vi "Minimum Gas Flow (Set).vi"(6 "ISOBUS address":T4=-1 caption="ISOBUS address (-1)", 8 "error in":errorcluster, 9 "Unit":T1, 10 "Min Flow":dbl caption="Minimum Gas Flow" min=0.0 max=20.0 step=0.1, 11 "Mercury Reference In":T5) -> (0 "error out":errorcluster, 2 "Response":T2, 3 "Mercury Reference Out":T5, 4 "Valid?":T3)   [LabVIEW 2019, in "Mercury iXX.lvlib" / "Auxiliary.lvlib"]
doc: "Set the current configuration for the minimum gas flow setting."
uses:
  Auxiliary.lvlib
  Controls/Mercury Reference.ctl
  CryoTUM_20210311/sub_vi-s/Equipment/Mercury iXX/Public/Controls/Comms Transport Layer.ctl
  Private/Controls/Query Dynamic Reference.ctl
  Controls/ISOBus Address.ctl
  Controls/Is Valid LED.ctl
  Controls/Response String.ctl
  Controls/Unit String.ctl
  Private/Controls/Command Verbs.ctl
  mercury/Mercury iXX.lvlib
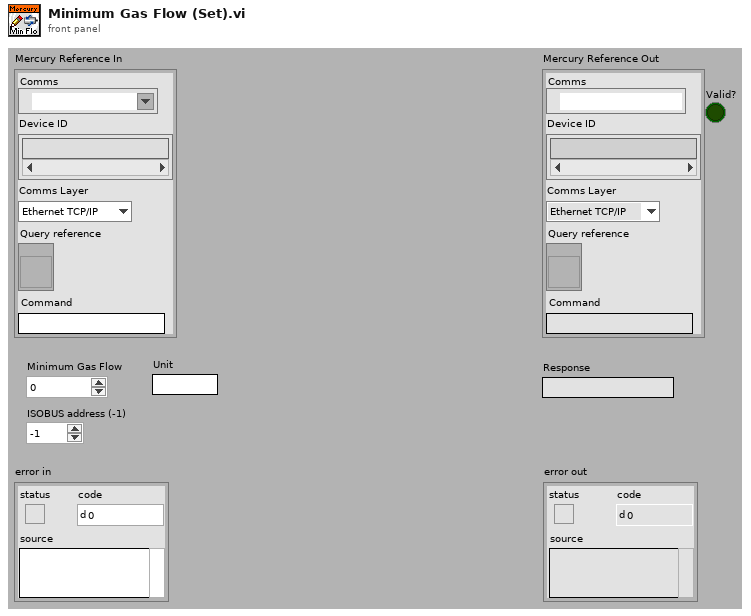
[diagram p1: front panel]
types:
  T1 = typedef "Mercury iXX.lvlib/Unit String.ctl" = string
  T2 = typedef "Mercury iXX.lvlib/Response String.ctl" = string
  T3 = typedef "Mercury iXX.lvlib/Is Valid LED.ctl" = bool
  T4 = typedef "Mercury iXX.lvlib/ISOBus Address.ctl" = i32
  T5 = typedef "Mercury iXX.lvlib/Mercury Reference.ctl" = cluster{"Comms":refnum<visa-resource-name>, "Device ID":string[], "Comms Layer":T6, "Command":string, "Query reference":T7}
  T6 = typedef "Mercury iXX.lvlib/Comms Transport Layer.ctl" = enum16{"Ethernet TCP/IP", "USB", "ISOBus - RS-232", "GPIB"}
  T7 = typedef "Mercury iXX.lvlib/Query Dynamic Reference.ctl" = refnum<vi>
  T8 = typedef "Mercury iXX.lvlib/Command Verbs.ctl" = string
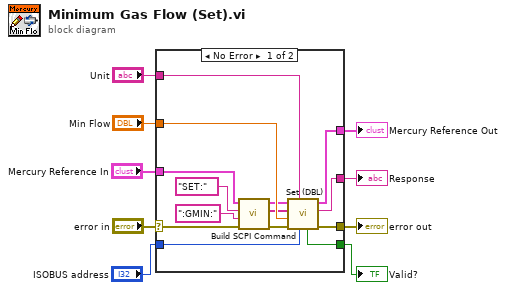
[diagram p0: block diagram]
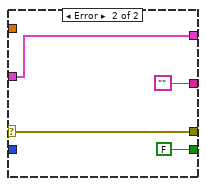
[diagram p2: hidden frame]
diagram:
  n1 = case shown="No Error" "error in" {
    selector: "error in" -> [w16 w26]
    tunnel: "Mercury Reference In" -> [w17 w27]
    tunnel: "ISOBUS address" -> [w23 _]
    tunnel: [w22 T3 FALSE ("Valid?")] -> w4
    tunnel: [w21 w26] -> w5
    tunnel: [w20 ""] -> w3
    tunnel: [w19 w27] -> w2
    tunnel: "Min Flow" -> [w18 _]
    tunnel: "Unit" -> [w10 _]
    frame No Error {
      n2 = call "Build SCPI Command.vi"("error in"=w16, "Noun(s)"=":GMIN:" ("Command"), "Verb"=T8 "SET:", "Mercury Reference In"=w17) -> ("error out"=w13:errorcluster, "SCPI Message(s)"=w15:string[], "Mercury Reference Out"=w14:T5)  [unwired: 5 out]
      n3 = call "Set (DBL).vi"("ISOBUS address"=w23, "Unit"=w10, "error in"=w13, "Command Value (Dbl)"=w18, "SCPI Message(s)"=w15, "Mercury Reference In"=w14) -> ("error out"=w21:errorcluster, "Response"=w20:T2, "Mercury Reference Out"=w19:T5, "Valid?"=w22:T3)  [unwired: 2 out]
    }
    frame Error {
    }
  }
  "Mercury Reference Out" <- w2
  "error out" <- w5
  "Valid?" <- w4
  "Response" <- w3
